vi "Close RF Sessions.vi"(0 "RF Subsystem Session Provider in":refnum<class "RF Subsystem Session Provider.lvclass">, 5 "TSM Context":T1, 11 "error in":errorcluster) -> (4 "RF Subsystem Session Provider out":refnum<class "RF Subsystem Session Provider.lvclass">, 15 "error out":errorcluster)   [LabVIEW 2023, in "RFFixtureCharact.RFPM.lvlib" / "RF Subsystem Session Provider.lvclass"]
uses:
  RF Subsystem Session Provider.lvclass
  <vilib>/NI_TestStand_SemiconductorModule/NI_TestStand_Semiconductor_Module.lvlibp/PinMap/General/SemiconductorModuleContext.ctl
  Common/Data Cache/Type Definitions/Dictionary Operation.ctl
  RF Subsystem Session Provider.lvclass/RF Subsystem Session Provider.ctl
  Common/RFCalAndFixtureCharact.Common.lvlib
  <vilib>/NI_TestStand_SemiconductorModule/NI_TestStand_Semiconductor_Module.lvlibp
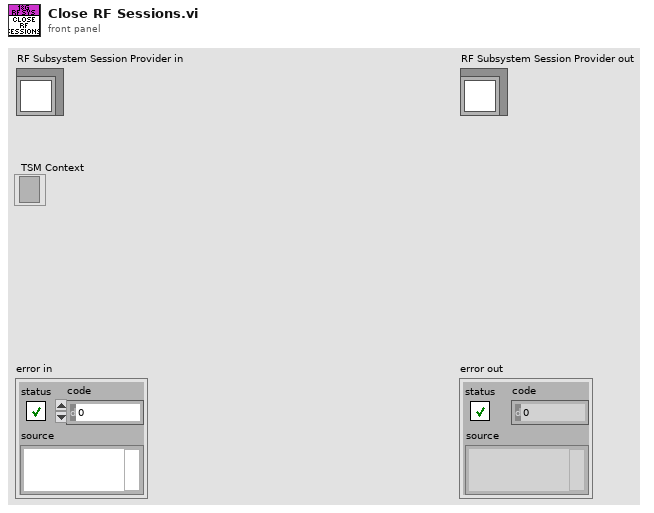
[diagram p1: front panel]
types:
  T1 = typedef "NI_TestStand_Semiconductor_Module.lvlibp/SemiconductorModuleContext.ctl" = refnum<k7>
  T2 = typedef "RFCalAndFixtureCharact.Common.lvlib/Dictionary Operation.ctl" = enum16{"Read", "Insert", "Remove", "Clear", "Get All", "Update"}
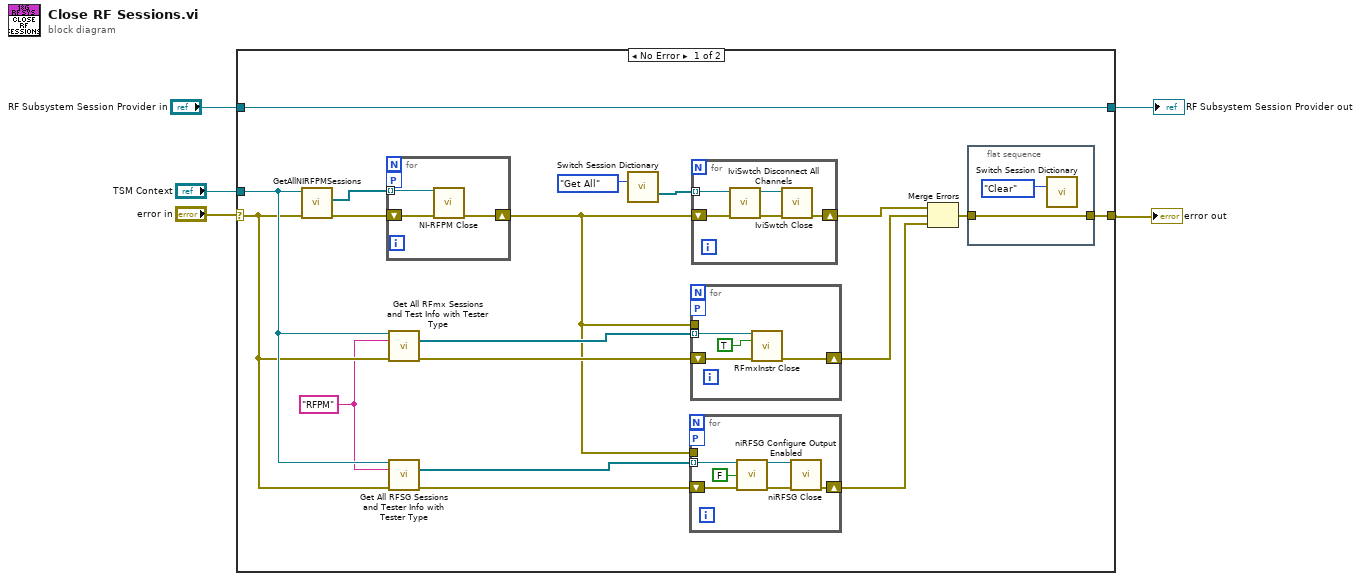
[diagram p0: block diagram]
diagram:
  n1 = case shown="No Error" "error in" {
    selector: "error in" -> [w14 w45]
    tunnel: [w9 w45] -> w5
    tunnel: "TSM Context" -> [w15 _]
    tunnel: "RF Subsystem Session Provider in" -> [w7 w44]
    tunnel: [w7 w44] -> w1
    frame No Error {
      w6 = "RFPM" ("Tester Type")
      n2 = call <vilib>:"GetAllNIRFPMSessions.vi"("error in (no error)"=w14, "Semiconductor Module Context"=w15) -> ("error out"=w19:errorcluster, "Instrument Sessions"=w18:refnum<k15>[])  [unwired: 7 in, 1 out]
      n3 = for {
        workers-P: _ -> [_]
        shift-right: [w32] -> w12
        shift-left: w19 -> [w31]
        tunnel: w18 -> [w33] mode=indexing
        n4 = call <instrlib>:"NI-RFPM Close.vi"("NI-5530 handle in"=w33, "error in"=w31) -> ("error out"=w32:errorcluster)  [unwired: 13 in]
      }
      n5 = call "Get All RFmx Sessions and Test Info with Tester Type.vi"("TSM Context In"=w15, "Tester Type"=w6, "error in"=w14) -> ("RFmx Sessions"=w23:refnum<k21>[], "error out"=w21:errorcluster)  [unwired: 8 in, 3 out]
      n6 = call "Get All RFSG Sessions and Tester Info with Tester Type.vi"("TSM Context In"=w15, "Tester Type"=w6, "error in"=w14) -> ("RFSG Sessions"=w22:refnum<k15>[], "error out"=w20:errorcluster)  [unwired: 8 in, 3 out]
      n7 = call "Switch Session Dictionary.vi"("Action"=Dictionary_Operation."Get All") -> ("All Ivi Switch Sessions Out"=w10:refnum<k15>[])  [unwired: 12 in, 2 out]
      n8 = for {
        tunnel: w22 -> [w36] mode=indexing
        workers-P: _ -> [_]
        shift-right: [w39] -> w16
        shift-left: w20 -> [w38]
        tunnel: w12 -> [_]
        n9 = call <instrlib>:"niRFSG Configure Output Enabled.vi"("instrument handle"=w36, "output enabled"=FALSE, "error in"=w38) -> ("instrument handle out"=w35:refnum<k15>, "error out"=w37:errorcluster)  [unwired: 11 in]
        n10 = call <instrlib>:"niRFSG Close.vi"("instrument handle"=w35, "error in"=w37) -> ("error out"=w39:errorcluster)  [unwired: 13 in]
      }
      n11 = for {
        tunnel: w23 -> [w43] mode=indexing
        workers-P: _ -> [_]
        shift-right: [w41] -> w17
        shift-left: w21 -> [w40]
        tunnel: w12 -> [_]
        n12 = call <vilib>:"RFmxInstr Close.vi"("Instrument Handle In"=w43, "Force Destroy? (F)"=TRUE, "error in (no error)"=w40) -> ("error out"=w41:errorcluster)  [unwired: 12 in]
      }
      n13 = for {
        tunnel: w10 -> [w28] mode=indexing
        shift-right: [w30] -> w13
        shift-left: w12 -> [w29]
        n14 = call <vilib>:"IviSwtch Disconnect All Channels.vi"("error in (no error)"=w29, "instrument handle"=w28) -> ("error out"=w27:errorcluster, "instrument handle out"=w26:refnum<k15>)  [unwired: 8 in]
        n15 = call <vilib>:"IviSwtch Close.vi"("error in (no error)"=w27, "instrument handle"=w26) -> ("error out"=w30:errorcluster)  [unwired: 9 in]
      }
      n16 = Merge Errors(w13, w17, w16) -> (w8:errorcluster)
      n17 = flat-sequence {
        tunnel: [w25] -> w9
        tunnel: w8 -> [w25]
        frame #0 {
          n18 = call "Switch Session Dictionary.vi"("Action"=Dictionary_Operation."Clear") -> ()  [unwired: 12 in, 3 out]
        }
      }
    }
    frame Error {
    }
  }
  "error out" <- w5
  "RF Subsystem Session Provider out" <- w1
